vi "TapeMonitor.vi"() -> ()   [LabVIEW 2011]
uses:
  GUI_Template/GUI_master/tcp_new_data_event.ctl
  GUI_Template/GUI_master/tcp new data cluster.ctl
  <vilib>/vision/Image Controls.llb/IMAQ Image.ctl
  <vilib>/vision/NI_Vision_Development_Module.lvlib
  <vilib>/Analysis/NI_AALBase.lvlib
panel:
  out "x-y":dbl
  out "sqrt(x)":dbl=0.9039278031128191
  out "fitness":dbl=0.7483901847989424
  out "area symmetry":dbl=0.8170854732403674
  out "standard deviation":dbl=201.25170806728573 format="%0.2f"
  out "Array":dbl[](array[numeric])=[1257.0, 807.0, 1140.0, 1197.0]
  out "symmetry":dbl=0.8279313704277508
  out "Number of Particles":i32=4
  out "X":dbl[](array[numeric])=[162.55608591885442, 93.22552664188352, 85.6640350877193, 149.66499582289055]
  out "Y":dbl[](array[numeric])=[105.60700079554495, 113.13382899628253, 177.49561403508773, 177.60902255639098]
  in  "Font, Size & Style":T1={"Desired Font (Application)"=enum."Application Font", "[User-specified Font]"={"Font Name"="", "Size"=12, "Strikeout?"=FALSE, "Italic?"=FALSE, "Underline?"=FALSE, "Outline?"=FALSE, "Shadow?"=FALSE, "Bold?"=FALSE, "Rotation Angle"=0.0}, "Horizontal Alignment"=0, "Vertical Alignment"=0} {"Vertical Alignment" items=["Bottom", "Top", "Baseline"]; "Horizontal Alignment" items=["Left", "Center", "Right"]; "[User-specified Font]"."Rotation Angle" format="%.2f"}
  in  "Selection Values":T3(array[cluster])=[{"Measurement Parameter"=35, "Range Lower Value"=0.0, "Range Upper Value"=500.0, "Range"=TRUE, "Measurement Type"=FALSE}] {"Measurement Parameter" items=["Center of Mass X", "Center of Mass Y", "First Pixel X", "First Pixel Y", "Bounding Rect Left", "Bounding Rect Top", "Bounding Rect Right", "Bounding Rect Bottom", "Max Feret Diameter Start X", "Max Feret Diameter Start Y", "Max Feret Diameter End X", "Max Feret Diameter End Y", "Max Horiz. Segment Length Left", "Max Horiz. Segment Length Right", "Max Horiz. Segment Length Row", "-", "Bounding Rect Width", "Bounding Rect Height", "Bounding Rect Diagonal", "Perimeter", "Convex Hull Perimeter", "Holes' Perimeter", "Max Feret Diameter", "Equivalent Ellipse Major Axis", "Equivalent Ellipse Minor Axis", "Equivalent Ellipse Minor Axis (Feret)", "Equivalent Rect Long Side", "Equivalent Rect Short Side", "Equivalent Rect Diagonal", "Equivalent Rect Short Side (Feret)", "Average Horiz. Segment Length", "Average Vert. Segment Length", "Hydraulic Radius", "Waddel Disk Diameter", "-", "Area", "Holes' Area", "Particle & Holes' Area", "Convex Hull Area", "Image Area", "-", "Number of Holes", "Number of Horiz. Segments", "Number of Vert. Segments", "-", "Orientation", "Max Feret Diameter Orientation", "-", "% Area/Image Area", "% Area/(Particle & Holes' Area)", "Ratio of Equivalent Ellipse Axes", "Ratio of Equivalent Rect Sides", "-", "Elongation Factor", "Compactness Factor", "Heywood Circularity Factor", "Type Factor", "-", "Sum X", "Sum Y", "Sum XX", "Sum XY", "Sum YY", "Sum XXX", "Sum XXY", "Sum XYY", "Sum YYY", "-", "Moment of Inertia XX", "Moment of Inertia XY", "Moment of Inertia YY", "Moment of Inertia XXX", "Moment of Inertia XXY", "Moment of Inertia XYY", "Moment of Inertia YYY", "Norm. Moment of Inertia XX", "Norm. Moment of Inertia XY", "Norm. Moment of Inertia YY", "Norm. Moment of Inertia XXX", "Norm. Moment of Inertia XXY", "Norm. Moment of Inertia XYY", "Norm. Moment of Inertia YYY", "Hu Moment 1", "Hu Moment 2", "Hu Moment 3", "Hu Moment 4", "Hu Moment 5", "Hu Moment 6", "Hu Moment 7"]}
  in  "Keep/Replace Value (Replace) 2":bool=TRUE
  out "image2":T4(plugin-control) caption="Mode1"
  in  "Size & Order # 2":T5={"X Size"=3, "Y Size"=3, "Order #"=4}
  in  "Range 2":cluster{"Lower value":sgl, "Upper value":sgl}={"Lower value"=128.0, "Upper value"=255.0} {"Upper value" format="%.2f"; "Lower value" format="%.2f"}
  in  "Size & Order #":T5={"X Size"=3, "Y Size"=3, "Order #"=4}
  in  "Range":cluster{"Lower value":sgl, "Upper value":sgl}={"Lower value"=48.0, "Upper value"=255.0} {"Upper value" format="%.2f"; "Lower value" format="%.2f"}
  in  "Keep/Replace Value (Replace)":bool=TRUE
  in  "gain::1":dbl caption="gain" min=0.0 max=12.0 format="%_4p"
  out "Histogram":T6(graph)
  out "image::1":T4(plugin-control) caption="Mode1"
  in  "exposure::1":dbl=0.01 caption="Exposure" min=0.0001 max=1.0 format="%_4p"
  in  "insert tag":bool=TRUE
  in  "stop":bool
  in  "trigger::1":bool caption="Trigger"
  in  "GUIdevice 1":string="StagingCapSideView"
  out "tcp data event":T7
  out "error IO 2":errorcluster
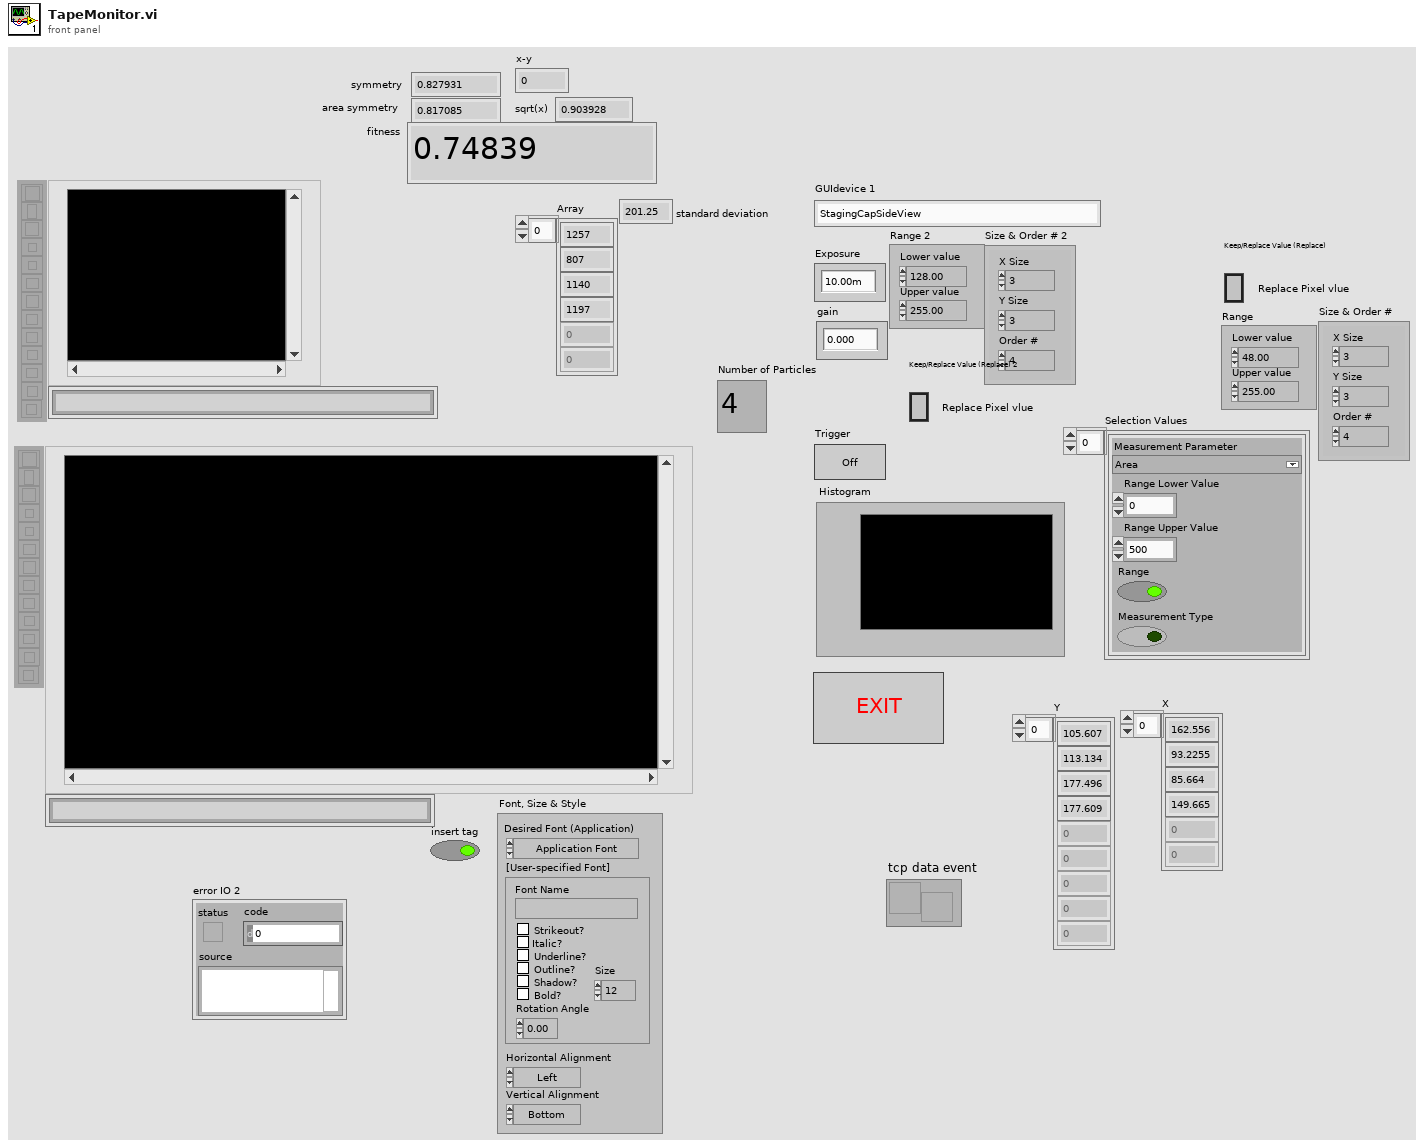
[diagram p1: front panel]
types:
  T1 = cluster{"Desired Font (Application)":enum16{"User-specified Font", "Application Font", "System Font", "Dialog Font"}, "[User-specified Font]":cluster{"Font Name":string, "Size":i16, "Strikeout?":bool, "Italic?":bool, "Underline?":bool, "Outline?":bool, "Shadow?":bool, "Bold?":bool, "Rotation Angle":dbl}, "Horizontal Alignment":i16, "Vertical Alignment":i16}
  T2 = typedef "Particle Parameters" = i32
  T3 = cluster{"Measurement Parameter":T2, "Range Lower Value":dbl, "Range Upper Value":dbl, "Range":bool, "Measurement Type":bool}[]
  T4 = typedef "IMAQ Image.ctl" = refnum<image>
  T5 = cluster{"X Size":i32, "Y Size":i32, "Order #":i32}
  T6 = cluster{"Starting Value":sgl, "Incremental Value":sgl, "Histogram":u32[]}
  T7 = typedef "tcp_new_data_event.ctl" = refnum<user-event>
  T8 = typedef "Image Type" = u32
  T9 = typedef "tcp new data cluster.ctl" = cluster{"EventEnum":enum16{"new data", "connection status update"}, "Device name":string}
  T10 = cluster{"Particle Measurements (Pixels)[0]":dbl, "Particle Measurements (Pixels)[1]":dbl, "Particle Measurements (Pixels)[2]":dbl, "Particle Measurements (Pixels)[3]":dbl}
  T11 = cluster{"Particle Measurements (Pixels)[0]":dbl, "Particle Measurements (Pixels)[1]":dbl}
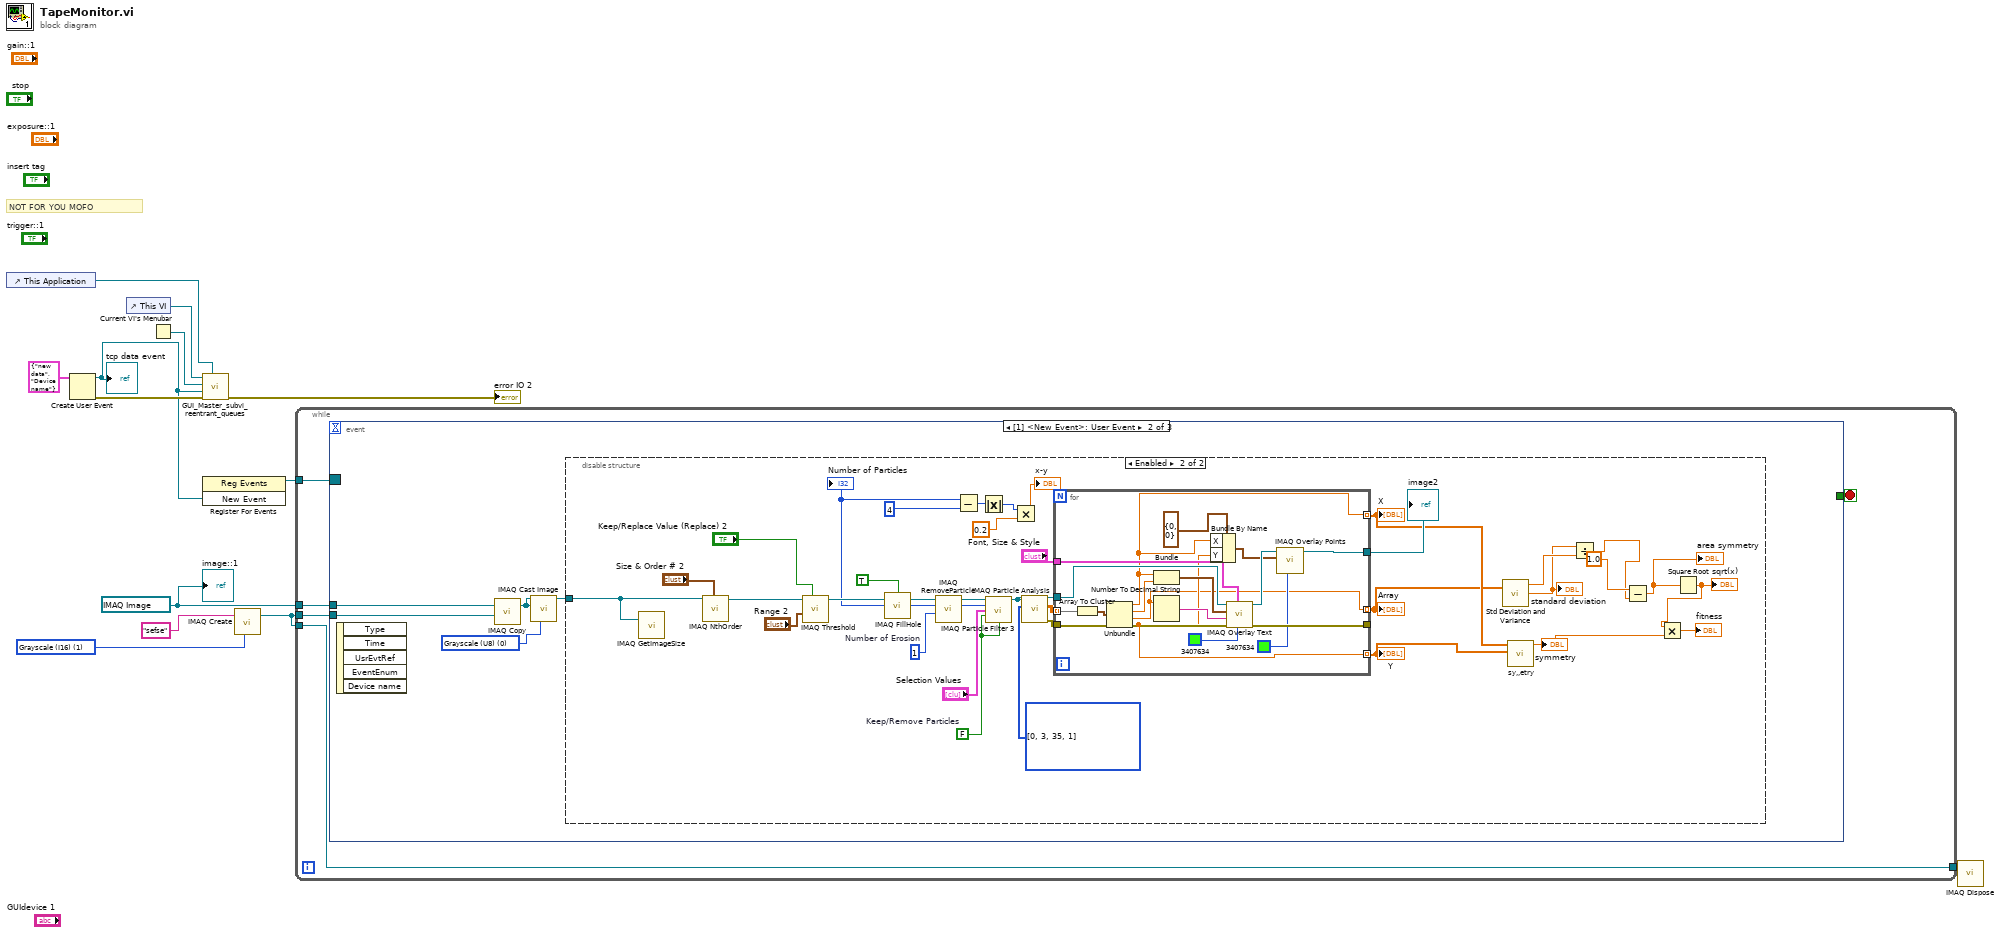
[diagram p0: block diagram]
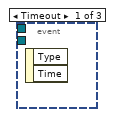
[diagram p2: hidden frame]
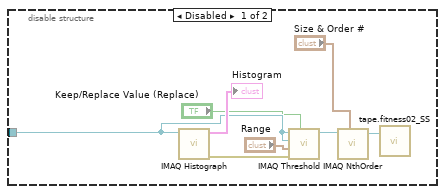
[diagram p3: hidden frame]
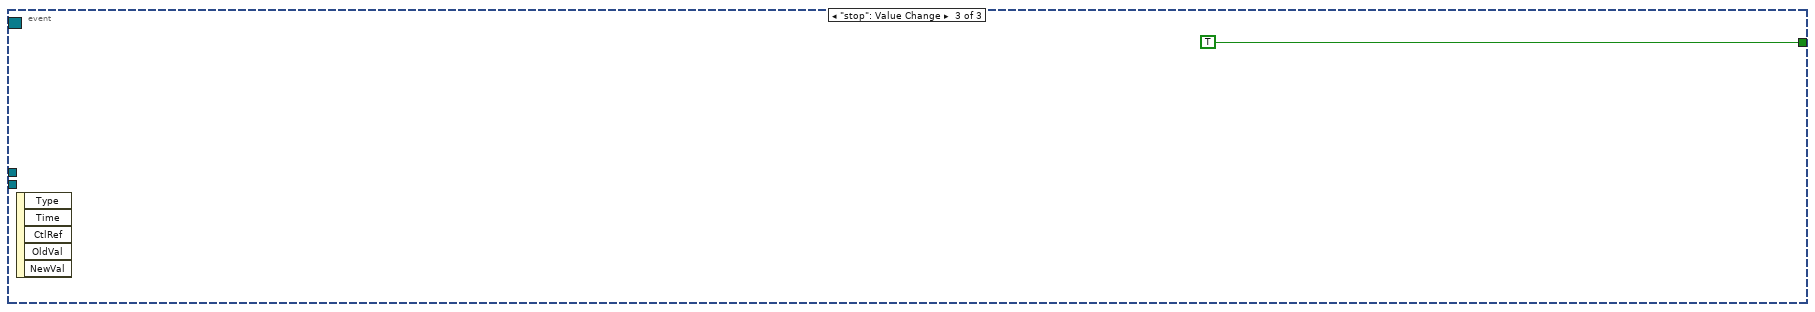
[diagram p4: hidden frame]
diagram:
  w5 = T8 1 items=["Grayscale (U8)", "Grayscale (I16)", "Grayscale (SGL)", "Complex (CSG)", "RGB (U32)", "HSL (U32)", "RGB (U64)", "Grayscale (U16)"] ("Image Type")
  w1 = T4 refnum ("New Image")
  # "NOT FOR YOU MOFO"
  n1 = control-ref of="This Application"() -> (w8:refnum<vi>)
  n2 = Create User Event(user event datatype=T9 {"EventEnum"=enum."new data", "Device name"="Device name"} ("New Event")) -> (user event=w6:refnum<user-event>, error out=w9:errorcluster)  [unwired: 1 in]
  "tcp data event" <- w6
  n3 = control-ref of="This VI"() -> (w12:refnum<vi>)
  n4 = Current VI's Menubar() -> (w11:refnum<k9>)
  n5 = call "GUI_Master_subvi_reentrant_queues.vi"("This Application"=w8, "error in (no error)"=w9, "tcp data event"=w6, "Caller menu reference"=w11, "Caller VI ref"=w12) -> ("error out"=→"error IO 2":errorcluster)  [unwired: 6 in]
  n6 = register-events(w6) -> (reference out=w7:refnum<event-registration>)  [unwired: 2 in, 1 out]
  n7 = call "IMAQ Create"("Image Name"="sefse", "Image Type"=w5) -> ("New Image"=w3:T4)  [unwired: 3 in, 1 out]
  n8 = while {
    tunnel: w7 -> [w17]
    tunnel: w1 -> [w16]
    tunnel: w3 -> [w15]
    tunnel: w3 -> [w14]
    tunnel: [w14] -> w2
    stop <- w18 stop-if-true
    n9 = event shown="[1] <New Event>: User Event" {
      selector: w17 -> [_ _ _]
      dyn-events: _ -> [_ _ _]
      timeout: _ -> [_ _ _]
      tunnel: [_ _ TRUE] -> w18
      tunnel: w16 -> [_ w22 _]
      tunnel: w15 -> [_ w23 _]
      event Timeout {
        n10 = event-data() -> ()  [unwired: 1 in, 2 out]
      }
      event User Event {
        w19 = T8 0 items=["Grayscale (U8)", "Grayscale (I16)", "Grayscale (SGL)", "Complex (CSG)", "RGB (U32)", "HSL (U32)", "RGB (U64)", "Grayscale (U16)"] ("Image Type")
        n11 = event-data() -> ()  [unwired: 1 in, 5 out]
        n12 = call "IMAQ Copy"("Image Dst"=w23, "Image Src"=w22) -> ("Image Dst Out"=w21:T4)  [unwired: 4 in, 1 out]
        n13 = call "IMAQ Cast Image"("Image Type"=w19, "Image Dst"=w21, "Image Src"=w21) -> ("Image Dst Out"=w20:T4)  [unwired: 7 in, 1 out]
        n14 = disable-structure shown="Enabled" {
          disable-tunnel: w20 -> [w29 w49]
          frame Disabled {
            n15 = call "IMAQ Histograph"("Image"=w29) -> ("error out"=w30:errorcluster, "Histogram Graph"=→"Histogram":T6)  [unwired: 7 in, 2 out]
            n16 = call "IMAQ Threshold"("Keep/Replace Value (Replace)"="Keep/Replace Value (Replace)", "error in (no error)"=w30, "Range"="Range", "Image Dst"=w29, "Image Src"=w29) -> ("Image Dst Out"=w26:T4)  [unwired: 5 in, 1 out]
            n17 = call "IMAQ NthOrder"("Image Src"=w26, "Size & Order #"="Size & Order #") -> ("Image Dst Out"=w25:T4)  [unwired: 5 in, 1 out]
            n18 = call "tape.fitness02_SS.vi"("New Image"=w25) -> ()  [unwired: 2 in]
          }
          frame Enabled {
            w51 = T2[] [0, 3, 35, 1] items=["Center of Mass X", "Center of Mass Y", "First Pixel X", "First Pixel Y", "Bounding Rect Left", "Bounding Rect Top", "Bounding Rect Right", "Bounding Rect Bottom", "Max Feret Diameter Start X", "Max Feret Diameter Start Y", "Max Feret Diameter End X", "Max Feret Diameter End Y", "Max Horiz. Segment Length Left", "Max Horiz. Segment Length Right", "Max Horiz. Segment Length Row", "-", "Bounding Rect Width", "Bounding Rect Height", "Bounding Rect Diagonal", "Perimeter", "Convex Hull Perimeter", "Holes' Perimeter", "Max Feret Diameter", "Equivalent Ellipse Major Axis", "Equivalent Ellipse Minor Axis", "Equivalent Ellipse Minor Axis (Feret)", "Equivalent Rect Long Side", "Equivalent Rect Short Side", "Equivalent Rect Diagonal", "Equivalent Rect Short Side (Feret)", "Average Horiz. Segment Length", "Average Vert. Segment Length", "Hydraulic Radius", "Waddel Disk Diameter", "-", "Area", "Holes' Area", "Particle & Holes' Area", "Convex Hull Area", "Image Area", "-", "Number of Holes", "Number of Horiz. Segments", "Number of Vert. Segments", "-", "Orientation", "Max Feret Diameter Orientation", "-", "% Area/Image Area", "% Area/(Particle & Holes' Area)", "Ratio of Equivalent Ellipse Axes", "Ratio of Equivalent Rect Sides", "-", "Elongation Factor", "Compactness Factor", "Heywood Circularity Factor", "Type Factor", "-", "Sum X", "Sum Y", "Sum XX", "Sum XY", "Sum YY", "Sum XXX", "Sum XXY", "Sum XYY", "Sum YYY", "-", "Moment of Inertia XX", "Moment of Inertia XY", "Moment of Inertia YY", "Moment of Inertia XXX", "Moment of Inertia XXY", "Moment of Inertia XYY", "Moment of Inertia YYY", "Norm. Moment of Inertia XX", "Norm. Moment of Inertia XY", "Norm. Moment of Inertia YY", "Norm. Moment of Inertia XXX", "Norm. Moment of Inertia XXY", "Norm. Moment of Inertia XYY", "Norm. Moment of Inertia YYY", "Hu Moment 1", "Hu Moment 2", "Hu Moment 3", "Hu Moment 4", "Hu Moment 5", "Hu Moment 6", "Hu Moment 7"] ("Pixel Measurements")
            w58 = FALSE  # Keep/Remove Particles
            w60 = 1  # Number of Erosion
            n19 = call "IMAQ GetImageSize"("Image"=w49) -> ()  [unwired: 3 in, 3 out]
            n20 = call "IMAQ NthOrder"("Image Src"=w49, "Size & Order #"="Size & Order # 2") -> ("Image Dst Out"=w66:T4)  [unwired: 5 in, 1 out]
            n21 = call "IMAQ Threshold"("Keep/Replace Value (Replace)"="Keep/Replace Value (Replace) 2", "Range"="Range 2", "Image Src"=w66) -> ("Image Dst Out"=w62:T4)  [unwired: 7 in, 1 out]
            n22 = call "IMAQ FillHole"("Image Src"=w62, "Connectivity 4/8 (8)"=TRUE) -> ("Image Dst Out"=w61:T4)  [unwired: 2 in, 3 out]
            n23 = call "IMAQ RemoveParticle"("Number of Erosion"=w60, "Image Src"=w61) -> ("Image Dst Out"=w57:T4)  [unwired: 5 in, 4 out]
            n24 = call "IMAQ Particle Filter 3"("Image Src"=w57, "Selection Values"="Selection Values", "Keep/Remove Particles (F)"=w58, "Fill Holes? (F)"=w58) -> ("Image Dst Out"=w52:T4, "Number of Particles"=w37:i32)  [unwired: 5 in, 5 out]
            "Number of Particles" <- w37
            n25 = Subtract(x=w37, y=4) -> (x-y=w35:i32)
            n26 = Absolute Value(x=w35) -> (abs(x)=w34:i32)
            n27 = Multiply(x=w34, y=0.2) -> (x*y=→"x-y":dbl)
            n28 = call "IMAQ Particle Analysis"("Pixel Measurements"=w51, "Image"=w52) -> ("error out"=w53:errorcluster, "Particle Measurements (Pixels)"=w55:dbl[][])  [unwired: 3 in, 5 out]
            n29 = for {
              tunnel: w53 -> [w84]
              tunnel: [w83] -> _
              tunnel: [w73] -> w50
              tunnel: w52 -> [w80]
              tunnel: "Font, Size & Style" -> [w76]
              tunnel: w55 -> [w75] mode=indexing
              tunnel: [w69] -> w47 mode=indexing
              tunnel: [w68] -> w48 mode=indexing
              tunnel: [w67] -> w46 mode=indexing
              n30 = Array To Cluster(array=w75) -> (cluster=w79:T10)
              n31 = Unbundle(w79) -> ("Particle Measurements (Pixels)[0]"=w69:dbl, "Particle Measurements (Pixels)[1]"=w78:dbl, "Particle Measurements (Pixels)[2]"=w67:dbl, "Particle Measurements (Pixels)[3]"=w68:dbl)
              n32 = Bundle("Particle Measurements (Pixels)[0]"=w69, "Particle Measurements (Pixels)[1]"=w78) -> (w77:T11)  [unwired: 1 out]
              n33 = Number To Decimal String(number=w67) -> (decimal integer string=w82:string)  [unwired: 1 out]
              n34 = Bundle By Name(cluster=cluster{"X":i32, "Y":i32} {"X"=0, "Y"=0} ("Point"), "X"=w69, "Y"=w68) -> (w70:cluster{"X":i32, "Y":i32})
              n35 = call "IMAQ Overlay Text"("Text Color (black)"=u32 3407634, "Font, Size & Style"=w76, "error in (no error)"=w84, "String"=w82, "Origin"=w77, "Image"=w80) -> ("error out"=w83:errorcluster, "Image Out"=w74:T4)  [unwired: 2 in, 2 out]
              n36 = call "IMAQ Overlay Points"("Color"=u32 3407634 ("Text Color (black)"), "Point"=w70, "Image"=w74) -> ("Image Out"=w73:T4)  [unwired: 7 in, 1 out]
            }
            "image2" <- w50
            "Y" <- w48
            "X" <- w47
            "Array" <- w46
            n37 = call <vilib>:"Std Deviation and Variance.vi"("X"=w46) -> ("mean"=w45:dbl, "standard deviation"=w44:dbl)  [unwired: 1 in, 1 out]
            "standard deviation" <- w44
            n38 = call "sy,,etry.vi"("Array 2"=w48, "Array"=w47) -> ("x-y 3"=w41:dbl)  [unwired: 9 in]
            "symmetry" <- w41
            n39 = Divide(x=w44, y=w45) -> (x/y=w42:dbl)
            n40 = Subtract(x=1.0 ("x/y"), y=w42) -> (x-y=w39:dbl)
            "area symmetry" <- w39
            n41 = Square Root(x=w39) -> (sqrt(x)=w38:dbl)
            "sqrt(x)" <- w38
            n42 = Multiply(x=w38, y=w41) -> (x*y=→"fitness":dbl)
          }
        }
      }
      event "stop": Value Change {
        n43 = event-data() -> ()  [unwired: 1 in, 5 out]
      }
    }
  }
  n44 = call "IMAQ Dispose"("Image"=w2) -> ()  [unwired: 5 in, 1 out]
  "image::1" <- w1
